vi "VNA Start Run.vi"(8 "error in (no error)":errorcluster, 11 "LibreVNA in":refnum<class "LibreVNA.lvclass">) -> (0 "error out":errorcluster, 1 "Is Running":bool, 3 "LibreVNA out":refnum<class "LibreVNA.lvclass">)   [LabVIEW 2023, in "LibreVNA.lvclass"]
uses:
  LibreVNA.lvclass
  LibreVNA.lvclass/LibreVNA.ctl
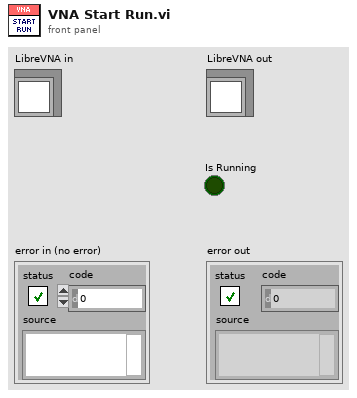
[diagram p1: front panel]
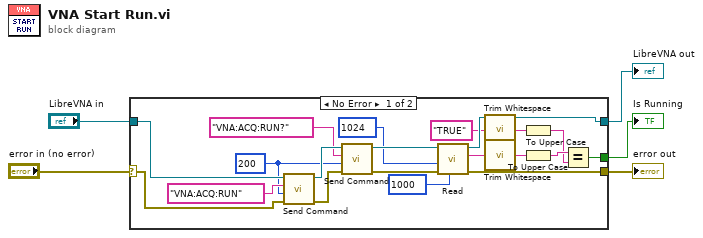
[diagram p0: block diagram]
diagram:
  n1 = case shown="No Error" "error in (no error)" {
    selector: "error in (no error)" -> [w23 w27]
    tunnel: [w10 w27] -> w4
    tunnel: [w17 w26] -> w2
    tunnel: "LibreVNA in" -> [w25 w26]
    tunnel: [w11 _] -> w1
    frame No Error {
      w19 = u32 200 ("command delay (ms)")
      n2 = call-dynamic "Send Command.vi"("error in (no error)"=w23, "command delay (ms)"=w19, "Command"="VNA:ACQ:RUN", "LibreVNA in"=w25) -> ("error out"=w21:errorcluster, "LibreVNA out"=w22:refnum<class "LibreVNA.lvclass">)  [unwired: 5 in, 1 out]
      n3 = call-dynamic "Send Command.vi"("error in (no error)"=w21, "command delay (ms)"=w19, "Command"="VNA:ACQ:RUN?", "LibreVNA in"=w22) -> ("error out"=w15:errorcluster, "LibreVNA out"=w18:refnum<class "LibreVNA.lvclass">)  [unwired: 5 in, 1 out]
      n4 = call-dynamic "Read.vi"("timeout ms (5000)"=1000, "error in (no error)"=w15, "bytes to read"=1024, "LibreVNA in"=w18) -> ("error out"=w10:errorcluster, "Recv Buffer"=w13:string, "LibreVNA out"=w17:refnum<class "LibreVNA.lvclass">)  [unwired: 5 in]
      n5 = call <vilib>:"Trim Whitespace.vi"("string"="TRUE" ("y")) -> ("trimmed string"=w6:string)  [unwired: 1 in]
      n6 = call <vilib>:"Trim Whitespace.vi"("string"=w13) -> ("trimmed string"=w9:string)  [unwired: 1 in]
      n7 = To Upper Case(1:w6) -> (0:w7:string)
      n8 = To Upper Case(1:w9) -> (0:w8:string)
      n9 = Equal?(x=w8, y=w7) -> (x = y?=w11:bool)
    }
    frame Error {
    }
  }
  "error out" <- w4
  "LibreVNA out" <- w2
  "Is Running" <- w1
